vi "GOOP_Library_Item_OnCommand.vi"(10 "Command Tag":string, 11 "Object":u64) -> ()   [LabVIEW 2020]
uses:
  SubVIs/GOOP_UMLEditor_CallMainAction.ctl
  ClassProviders/Provider_BaseClassInterface/ClassWriter_class/ClassWriter.lvclass
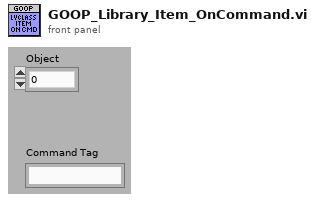
[diagram p1: front panel]
types:
  T1 = typedef "GOOP_UMLEditor_CallMainAction.ctl" = enum16{"OpenUmlEditor", "ReverseEngineering:WholeProject", "ReverseEngineering:OneClass", "ReverseEngineering:OneVI", "ShowInStateDiagram:OneVI", "OpenUMLFile"}
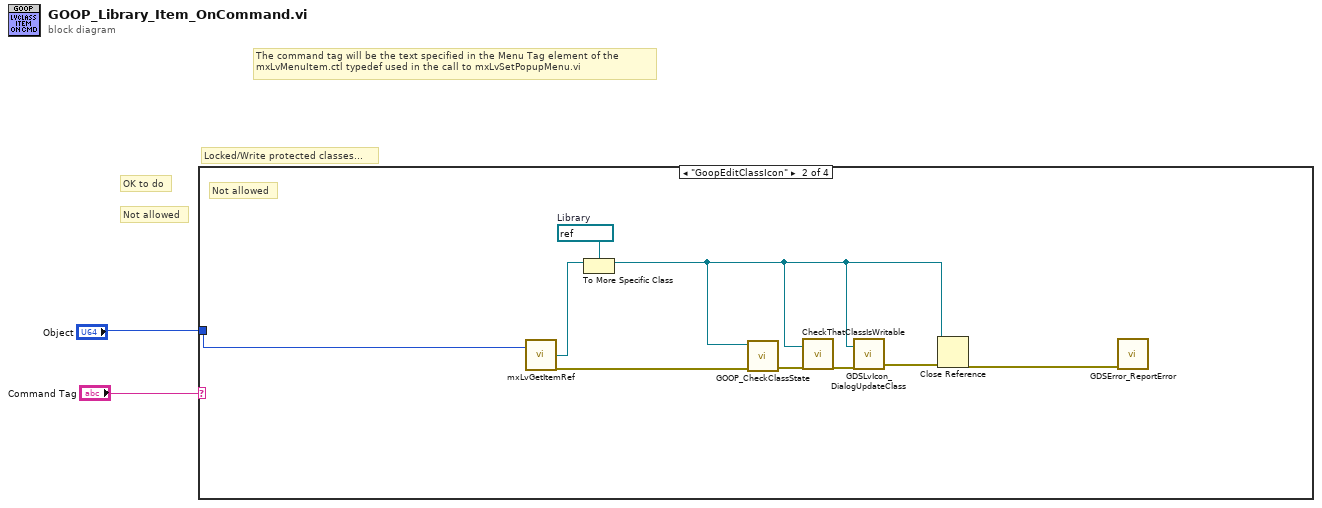
[diagram p0: block diagram]
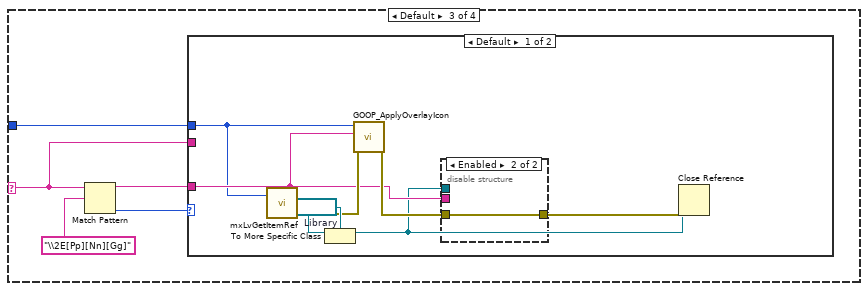
[diagram p3: hidden frame]
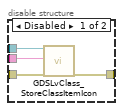
[diagram p4: hidden frame]
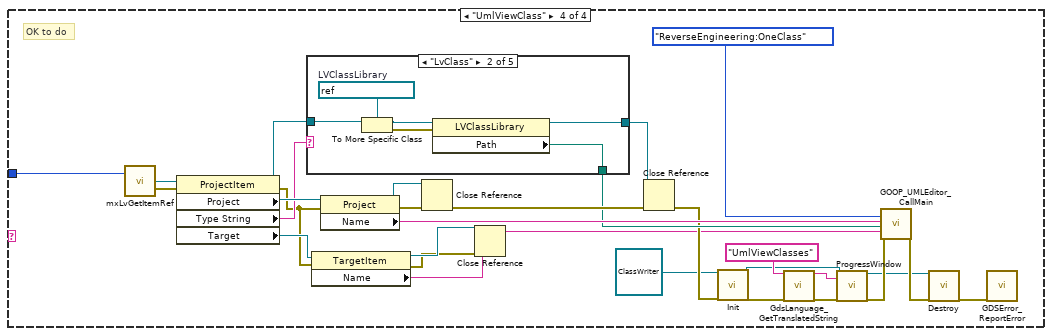
[diagram p6: hidden frame]
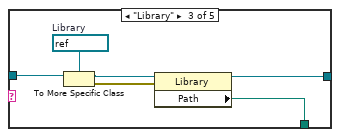
[diagram p8: hidden frame]
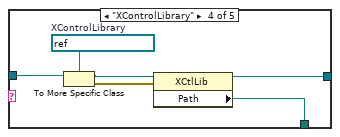
[diagram p9: hidden frame]
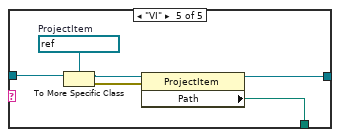
[diagram p10: hidden frame]
diagram:
  # "Not allowed"
  # "OK to do"
  # "Locked/Write protected classes..."
  # "The command tag will be the text specified in the Menu Tag element of the \nmxLvMenuItem.ctl typedef used in the call to mxLvSetPopupMenu.vi"
  n1 = case shown="\"GoopEditClassIcon\"" "Command Tag" {
    selector: "Command Tag" -> [_ _ w14 _]
    tunnel: "Object" -> [_ w10 w15 w35]
    frame "False" {
    }
    frame "GoopEditClassIcon" {
      w11 = refnum<vi> refnum  # Library
      # "Not allowed"
      n2 = call <resource>:"mxLvGetItemRef.vi"("Item"=w10) -> ("Item Refnum"=w9:refnum<vi>, "error out"=w4:errorcluster)  [unwired: 1 in, 1 out]
      n3 = To More Specific Class(target class=w11, reference=w9) -> (specific class reference=w3:refnum<vi>)  [unwired: 1 in, 1 out]
      n4 = call "GOOP_CheckClassState.vi"("error in"=w4, "Library Refnum"=w3) -> ("error out"=w5:errorcluster)  [unwired: 9 in]
      n5 = call "CheckThatClassIsWritable.vi"("Library Refnum"=w3, "error in (no error)"=w5) -> ("error out"=w6:errorcluster)  [unwired: 16 in, 1 out]
      n6 = call "GDSLvIcon_DialogUpdateClass.vi"("ClassPath(FilePath/ProjectTreePath/LvCLassRef)"=w3, "error in (no error)"=w6) -> ("error out"=w8:errorcluster)  [unwired: 14 in, 3 out]
      n7 = Close Reference(reference=w3, error in (no error)=w8) -> (error out=w7:errorcluster)
      n8 = call "GDSError_ReportError.vi"("error in (no error)"=w7) -> ()  [unwired: 18 in, 1 out]
    }
    frame Default {
      n9 = Match Pattern(string=w14, regular expression="\\2E[Pp][Nn][Gg]") -> (before substring=w12:string, offset past match=w13:i32)  [unwired: 1 in, 2 out]
      n10 = case shown="Default" w13 {
        tunnel: w15 -> [w18 _]
        tunnel: w14 -> [_ _]
        tunnel: w12 -> [w19 _]
        frame Default {
          w24 = refnum<vi> refnum  # Library
          n11 = call <resource>:"mxLvGetItemRef.vi"("Item"=w18) -> ("Item Refnum"=w23:refnum<vi>, "error out"=w22:errorcluster)  [unwired: 1 in, 1 out]
          n12 = To More Specific Class(target class=w24, reference=w23) -> (specific class reference=w17:refnum<vi>)  [unwired: 1 in, 1 out]
          n13 = call "GOOP_ApplyOverlayIcon.vi"("error in (no error)"=w22, "IconName(NoPngExtension)"=w19, "Object"=w18) -> ("error out"=w21:errorcluster)  [unwired: 8 in]
          n14 = disable-structure shown="Enabled" {
            disable-tunnel: w21 -> [w28 w29]
            disable-tunnel: [w27 w29] -> w20
            disable-tunnel: w19 -> [w26 _]
            disable-tunnel: w17 -> [w25 _]
            frame Disabled {
              n15 = call "GDSLvClass_StoreClassItemIcon.vi"("Library Refnum"=w25, "ClassItemIconName"=w26, "error in (no error)"=w28) -> ("error out"=w27:errorcluster)  [unwired: 15 in, 1 out]
            }
            frame Enabled {
            }
          }
          n16 = Close Reference(reference=w17, error in (no error)=w20) -> ()  [unwired: 1 out]
        }
        frame -1 {
        }
      }
    }
    frame "UmlViewClass" {
      # "OK to do"
      n17 = call <resource>:"mxLvGetItemRef.vi"("Item"=w35) -> ("Item Refnum"=w57:refnum<vi>, "error out"=w47:errorcluster)  [unwired: 1 in, 1 out]
      n18 = property class="ProjectItem"(reference=w57, error in=w47) -> (reference out=w51:refnum<vi>, error out=w30:errorcluster, "Project"=w56:refnum<vi>, "Type String"=w49:string, "Target"=w34:refnum<vi>)
      n19 = case shown="\"LvClass\"" w49 {
        tunnel: w51 -> [w59 w65 w71 w77 w83]
        tunnel: [w59 w61 w67 w73 w79] -> w50
        tunnel: [_ w60 w66 w72 w78] -> w48
        frame Default {
        }
        frame "LvClass" {
          w64 = refnum<vi> refnum  # LVClassLibrary
          n20 = To More Specific Class(target class=w64, reference=w65) -> (specific class reference=w63:refnum<vi>, error out=w62:errorcluster)  [unwired: 1 in]
          n21 = property class="LVClassLibrary"(reference=w63, error in=w62) -> (reference out=w61:refnum<vi>, "Path"=w60:path)  [unwired: 1 out]
        }
        frame "Library" {
          w70 = refnum<vi> refnum  # Library
          n22 = To More Specific Class(target class=w70, reference=w71) -> (specific class reference=w69:refnum<vi>, error out=w68:errorcluster)  [unwired: 1 in]
          n23 = property class="Library"(reference=w69, error in=w68) -> (reference out=w67:refnum<vi>, "Path"=w66:path)  [unwired: 1 out]
        }
        frame "XControlLibrary" {
          w76 = refnum<vi> refnum  # XControlLibrary
          n24 = To More Specific Class(target class=w76, reference=w77) -> (specific class reference=w75:refnum<vi>, error out=w74:errorcluster)  [unwired: 1 in]
          n25 = property class="XCtlLib"(reference=w75, error in=w74) -> (reference out=w73:refnum<vi>, "Path"=w72:path)  [unwired: 1 out]
        }
        frame "VI" {
          w82 = refnum<vi> refnum  # ProjectItem
          n26 = To More Specific Class(target class=w82, reference=w83) -> (specific class reference=w81:refnum<vi>, error out=w80:errorcluster)  [unwired: 1 in]
          n27 = property class="ProjectItem"(reference=w81, error in=w80) -> (reference out=w79:refnum<vi>, "Path"=w78:path)  [unwired: 1 out]
        }
      }
      n28 = property class="TargetItem"(reference=w34, error in=w30) -> (reference out=w32:refnum<vi>, error out=w31:errorcluster, "Name"=w33:string)
      n29 = property class="Project"(reference=w56, error in=w30) -> (reference out=w53:refnum<vi>, error out=w54:errorcluster, "Name"=w55:string)
      n30 = Close Reference(reference=w53, error in (no error)=w54) -> (error out=w52:errorcluster)
      n31 = Close Reference(reference=w32, error in (no error)=w31) -> ()  [unwired: 1 out]
      n32 = Close Reference(reference=w50, error in (no error)=w52) -> (error out=w43:errorcluster)
      n33 = call-dynamic "Init.vi"("ClassWriter in"=refnum<class "ClassWriter.lvclass"> refnum, "error in (no error)"=w43) -> ("ClassWriter out"=w38:refnum<class "ClassWriter.lvclass">, "error out"=w42:errorcluster)  [unwired: 16 in]
      n34 = call "GdsLanguage_GetTranslatedString.vi"("StringID(s)"="UmlViewClasses" ("Message(Exit)"), "error in (no error)"=w42) -> ("FirstStringOut"=w46:string, "error out"=w45:errorcluster)  [unwired: 14 in, 2 out]
      n35 = call-dynamic "ProgressWindow.vi"("ClassWriter in"=w38, "Message(Exit)"=w46, "error in (no error)"=w45) -> ("ClassWriter out"=w39:refnum<class "ClassWriter.lvclass">, "error out"=w41:errorcluster)  [unwired: 15 in]
      n36 = call "GOOP_UMLEditor_CallMain.vi"("Enum"=GOOP_UMLEditor_CallMainAction."ReverseEngineering:OneClass", "Project"=w55, "Class/VI-Path"=w48, "Target"=w33, "error in (no error)"=w41) -> ("error out"=w40:errorcluster)  [unwired: 14 in]
      n37 = call-dynamic "Destroy.vi"("ClassWriter.lvclass"=w39, "error in (no error)"=w40) -> ("error out"=w37:errorcluster)  [unwired: 17 in]
      n38 = call "GDSError_ReportError.vi"("error in (no error)"=w37) -> ()  [unwired: 18 in, 1 out]
    }
  }
